vi "checkChannelsCreated.vi"(8 "error in (no error)":errorcluster, 11 "Connection.NetworkStream in":refnum<class "Connection.NetworkStream.lvclass">) -> (0 "error out":errorcluster, 1 "outbound created":bool, 2 "inbound created":bool, 3 "Connection.NetworkStream out":refnum<class "Connection.NetworkStream.lvclass">)   [LabVIEW 2013, in "Connection.NetworkQueue_GOSPL.lvlib" / "Connection.NetworkStream.lvclass"]
uses:
  Connection.NetworkStream.lvclass
  Connection/Connection.lvclass
  Connection.NetworkStream.lvclass/Connection.NetworkStream.ctl
  <resource>/objmgr/ni.dex.rc
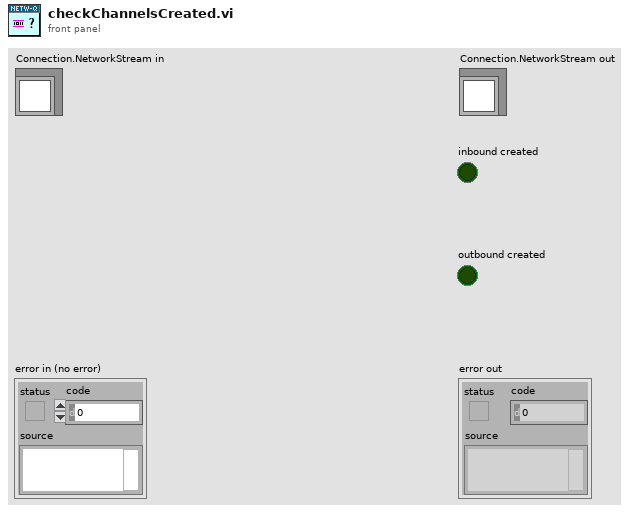
[diagram p1: front panel]
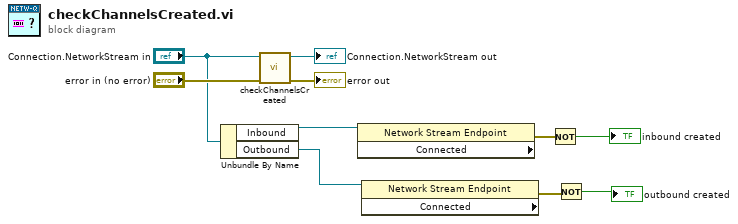
[diagram p0: block diagram]
diagram:
  n1 = Unbundle By Name("Connection.NetworkStream in") -> ("Inbound"=w6:refnum<k21>, "Outbound"=w5:refnum<k21>)
  n2 = call-parent "checkChannelsCreated.vi"("error in (no error)"="error in (no error)", "Connection in"="Connection.NetworkStream in") -> ("error out"=→"error out":errorcluster, "Connection out"=→"Connection.NetworkStream out":refnum<class "Connection.NetworkStream.lvclass">)  [unwired: 6 in, 2 out]
  n3 = property class="Network Stream Endpoint" props=["Connected"](reference=w6) -> (error out=w2:errorcluster)  [unwired: 1 in, 2 out]
  n4 = property class="Network Stream Endpoint" props=["Connected"](reference=w5) -> (error out=w4:errorcluster)  [unwired: 1 in, 2 out]
  n5 = Not(x=w2) -> (.not. x?=→"inbound created":bool)
  n6 = Not(x=w4) -> (.not. x?=→"outbound created":bool)
